vi "histerese_finite_state_machine.vi"() -> ()   [LabVIEW 2019]
panel:
  out "Fused":dbl
  in  "Tab Control":enum32{"Page 1", "Page 2"}(tab)
  in  "Pitot":dbl
  in  "Termico":dbl
  in  "Set point":dbl(slide) scale=2.0..20.0
  in  "stop":bool
  out "String":string
  in  "hist_min":dbl
  in  "hist_max":dbl
  out "Boolean":bool
  out "?":dbl
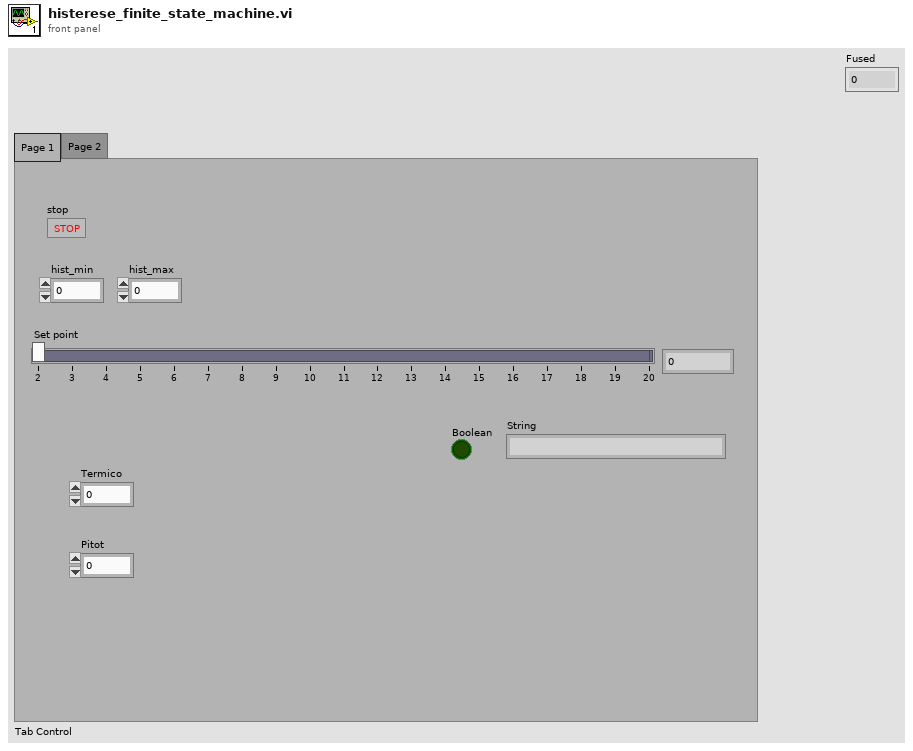
[diagram p1: front panel]
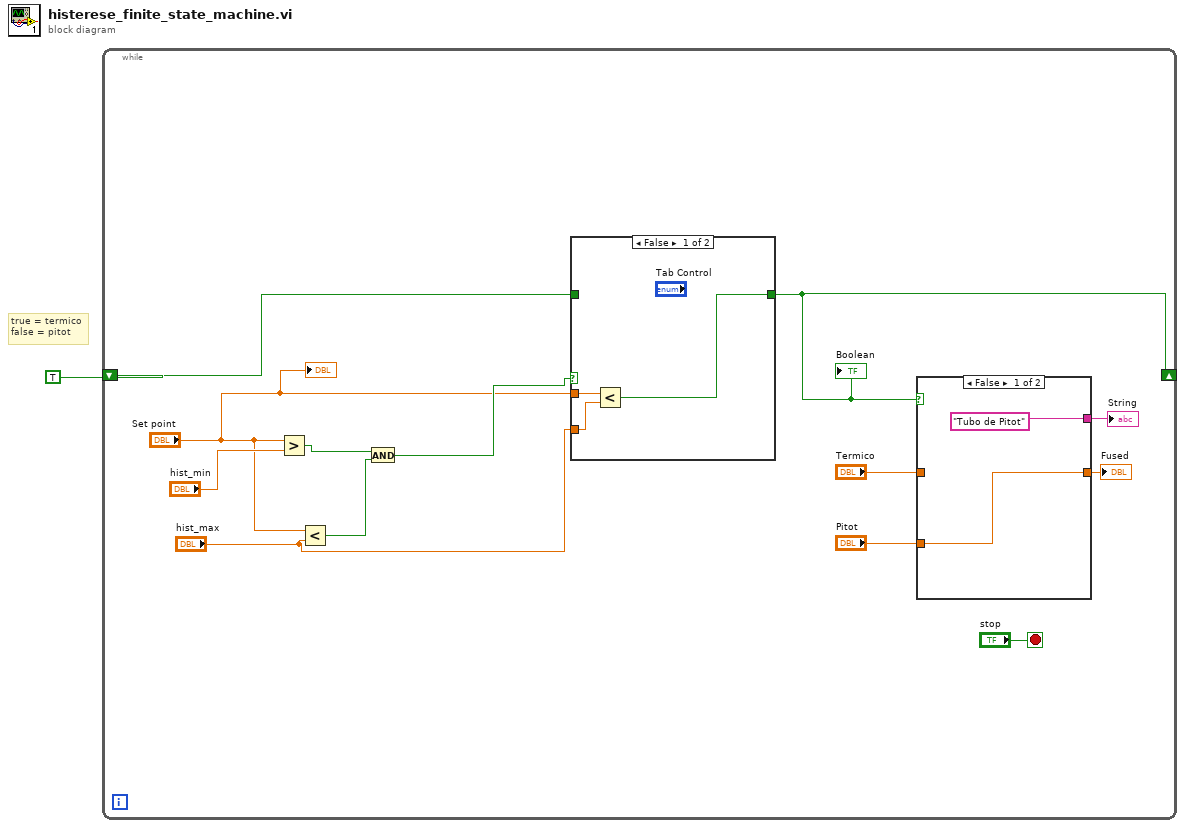
[diagram p0: block diagram]
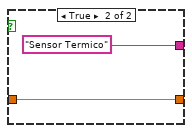
[diagram p2: hidden frame]
diagram:
  # "true = termico\nfalse = pitot"
  n1 = while {
    shift-right: [w9] -> _
    shift-left: TRUE ("Boolean") -> [w10]
    stop <- "stop" stop-if-true
    n2 = Greater?(x="Set point", y="hist_min") -> (0:w12:bool)
    n3 = Less?(x="Set point", y="hist_max") -> (x < y?=w13:bool)
    n4 = And(x=w12, y=w13) -> (x .and. y?=w11:bool)
    n5 = case shown="False" w11 {
      tunnel: w10 -> [_ w22]
      tunnel: [w19 w22] -> w9
      tunnel: "Set point" -> [w21 _]
      tunnel: "hist_max" -> [w20 _]
      frame False {
        n6 = Less?(x=w21, y=w20) -> (x < y?=w19:bool)
      }
      frame True {
      }
    }
    "Boolean" <- w9
    n7 = case shown="False" w9 {
      tunnel: ["Tubo de Pitot" "Sensor Termico"] -> w8
      tunnel: "Termico" -> [_ w17]
      tunnel: "Pitot" -> [w15 _]
      tunnel: [w15 w17] -> w2
      frame False {
      }
      frame True {
      }
    }
    "String" <- w8
    "Fused" <- w2
    "?" <- "Set point"
  }
